vi "Message type that caused error.vi"(11 "ErrorHandler JSON in":refnum<class "ErrorHandler JSON.lvclass">) -> (2 "Error in response to message type":T1, 3 "ErrorHandler JSON out":refnum<class "ErrorHandler JSON.lvclass">)   [LabVIEW 2020, in "wamplv.lvlib" / "ErrorHandler JSON.lvclass"]
uses:
  ErrorHandler JSON.lvclass
  TypeDefs/WAMP Message Codes.ctl
  wamplv.lvlib
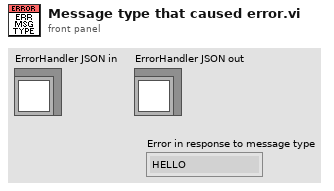
[diagram p1: front panel]
types:
  T1 = typedef "wamplv.lvlib/WAMP Message Codes.ctl" = enum8{"HELLO", "WELCOME", "CHALLENGE", "AUTHENTICATE", "ABORT", "GOODBYE", "ERROR", "PUBLISH", "PUBLISHED", "SUBSCRIBE", "SUBSCRIBED", "UNSUBSCRIBE", "UNSUBSCRIBED", "EVENT", "CALL", "RESULT", "REGISTER", "REGISTERED", "UNREGISTER", "UNREGISTERED", "INVOCATION", "YIELD"}
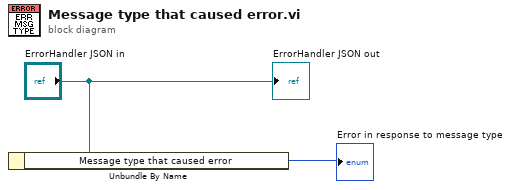
[diagram p0: block diagram]
diagram:
  n1 = Unbundle By Name("ErrorHandler JSON in") -> ("Message type that caused error"=→"Error in response to message type":T1)
  "ErrorHandler JSON out" <- "ErrorHandler JSON in"
